vi "UI Refresh.vi"(8 "error in (no error)":errorcluster, 11 "Controller in":refnum<class "Controller.lvclass">) -> (0 "error out":errorcluster, 3 "Controller out":refnum<class "Controller.lvclass">)   [LabVIEW 2013, in "SET Project Editor.lvlib" / "Controller.lvclass"]
uses:
  Controller.lvclass
  Controller.lvclass/Controller.ctl
  SET Project Data/Project Data Class/Project Data.lvclass
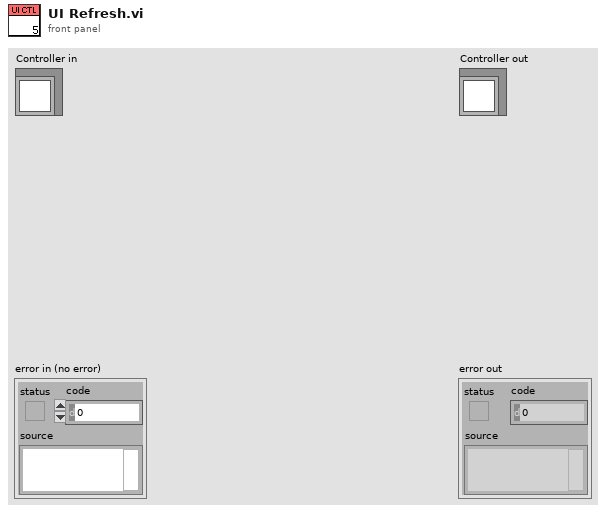
[diagram p1: front panel]
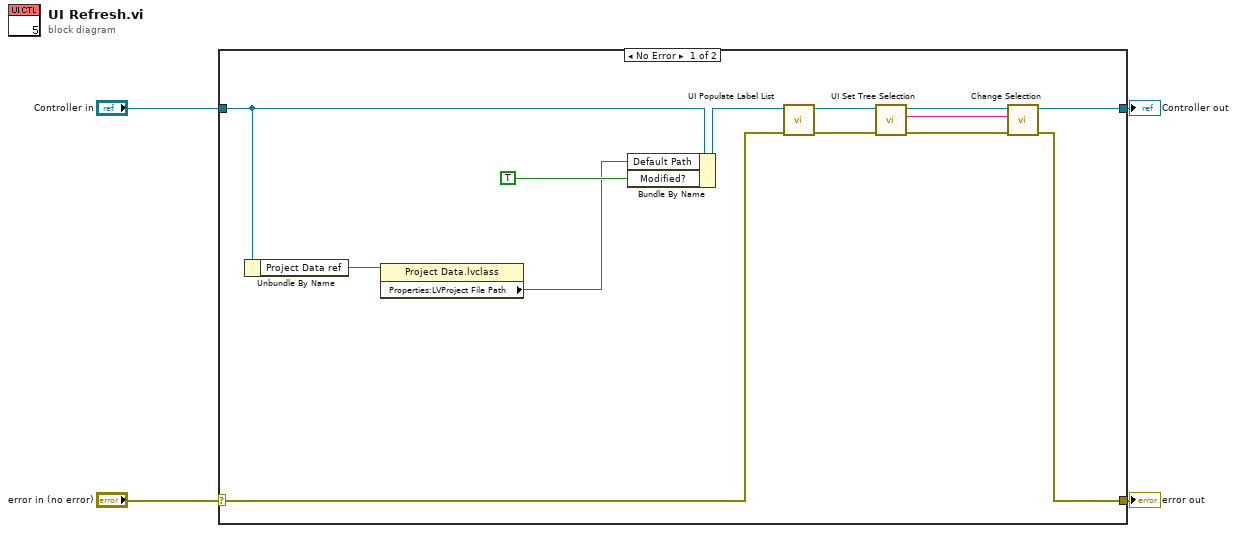
[diagram p0: block diagram]
diagram:
  n1 = case shown="No Error" "error in (no error)" {
    selector: "error in (no error)" -> [w6 w19]
    tunnel: [w8 w19] -> w3
    tunnel: [w9 w18] -> w1
    tunnel: "Controller in" -> [w10 w18]
    frame No Error {
      n2 = Unbundle By Name(w10) -> ("Project Data ref"=w5:refnum<data-value>)
      n3 = property class="Project Data.lvclass"(reference=w5) -> ("Properties:LVProject File Path"=w7:path)  [unwired: 1 in, 2 out]
      n4 = Bundle By Name(cluster=w10, "Default Path"=w7, "Modified?"=TRUE) -> (w16:refnum<class "Controller.lvclass">)
      n5 = call-dynamic "UI Populate Label List.vi"("error in (no error)"=w6, "Controller in"=w16) -> ("error out"=w14:errorcluster, "Controller out"=w15:refnum<class "Controller.lvclass">)  [unwired: 8 in]
      n6 = call-dynamic "UI Set Tree Selection.vi"("error in (no error)"=w14, "Controller in"=w15) -> ("error out"=w12:errorcluster, "Tag out"=w11:string, "Controller out"=w13:refnum<class "Controller.lvclass">)  [unwired: 7 in]
      n7 = call-dynamic "Change Selection.vi"("error in (no error)"=w12, "UID"=w11, "Controller in"=w13) -> ("error out"=w8:errorcluster, "Controller out"=w9:refnum<class "Controller.lvclass">)  [unwired: 7 in]
    }
    frame Error {
    }
  }
  "error out" <- w3
  "Controller out" <- w1
